vi "Simulated.vi"(9 "Stop Button":bool, 10 "Starting Temp":dbl, 11 "V Applied On?":bool) -> (3 "Temperature":dbl)   [LabVIEW 2012]
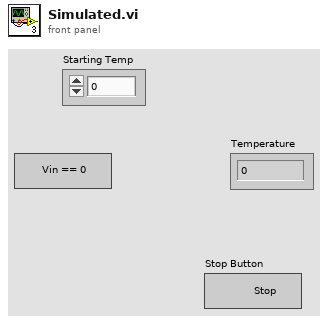
[diagram p1: front panel]
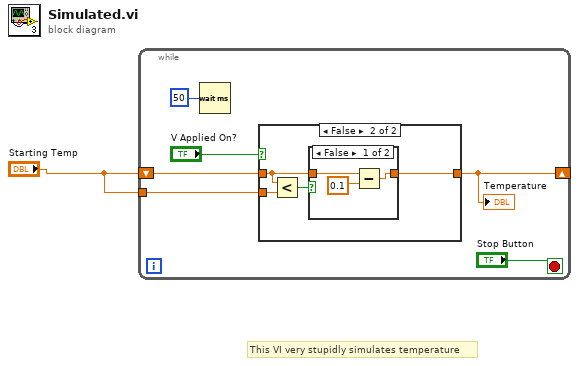
[diagram p0: block diagram]
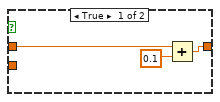
[diagram p2: hidden frame]
diagram:
  # "This VI very stupidly simulates temperature"
  n1 = while {
    shift-right: [w2] -> _
    shift-left: "Starting Temp" -> [w7]
    tunnel: "Starting Temp" -> [w5]
    stop <- "Stop Button" stop-if-true
    n2 = Wait (ms)(milliseconds to wait=u32 50) -> ()  [unwired: 1 out]
    n3 = case shown="False" "V Applied On?" {
      tunnel: w7 -> [w10 w13]
      tunnel: w5 -> [_ w12]
      tunnel: [w9 w14] -> w2
      frame True {
        n4 = Add(x=w10, y=0.1) -> (x+y=w9:dbl)
      }
      frame False {
        n5 = Less?(x=w13, y=w12) -> (x < y?=w11:bool)
        n6 = case shown="False" w11 {
          tunnel: w13 -> [w16 w18]
          tunnel: [w15 w18] -> w14
          frame False {
            n7 = Subtract(x=w16, y=0.1) -> (x-y=w15:dbl)
          }
          frame True {
          }
        }
      }
    }
    "Temperature" <- w2
  }
